vi "CRYSet Unicode Property Force Unicode Input.vi"(7 "Force Unicode Text (T)":bool, 8 "error in (no error)":errorcluster, 9 "String Control Reference":refnum<vi>) -> (2 "error out":errorcluster, 3 "String Control Reference":refnum<vi>)   [LabVIEW 2013]
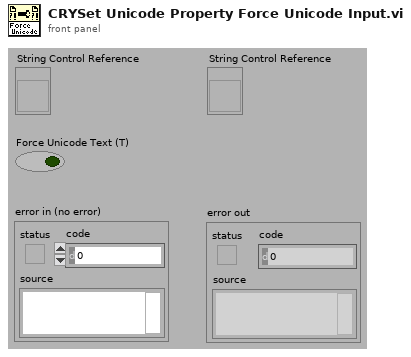
[diagram p1: front panel]
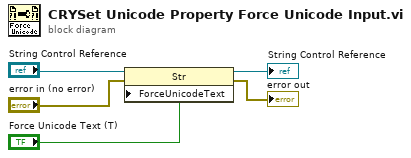
[diagram p0: block diagram]
diagram:
  n1 = property class="Str"(reference="String Control Reference", error in="error in (no error)", "ForceUnicodeText"="Force Unicode Text (T)") -> (reference out=→"String Control Reference":refnum<vi>, error out=→"error out":errorcluster)
